vi "vision messing around.vi"() -> ()   [LabVIEW 2010]
panel:
  out "Image Out 3":T1(plugin-control)
  out "Image Out 2":T1(plugin-control)
  in  "Stop (F)":bool
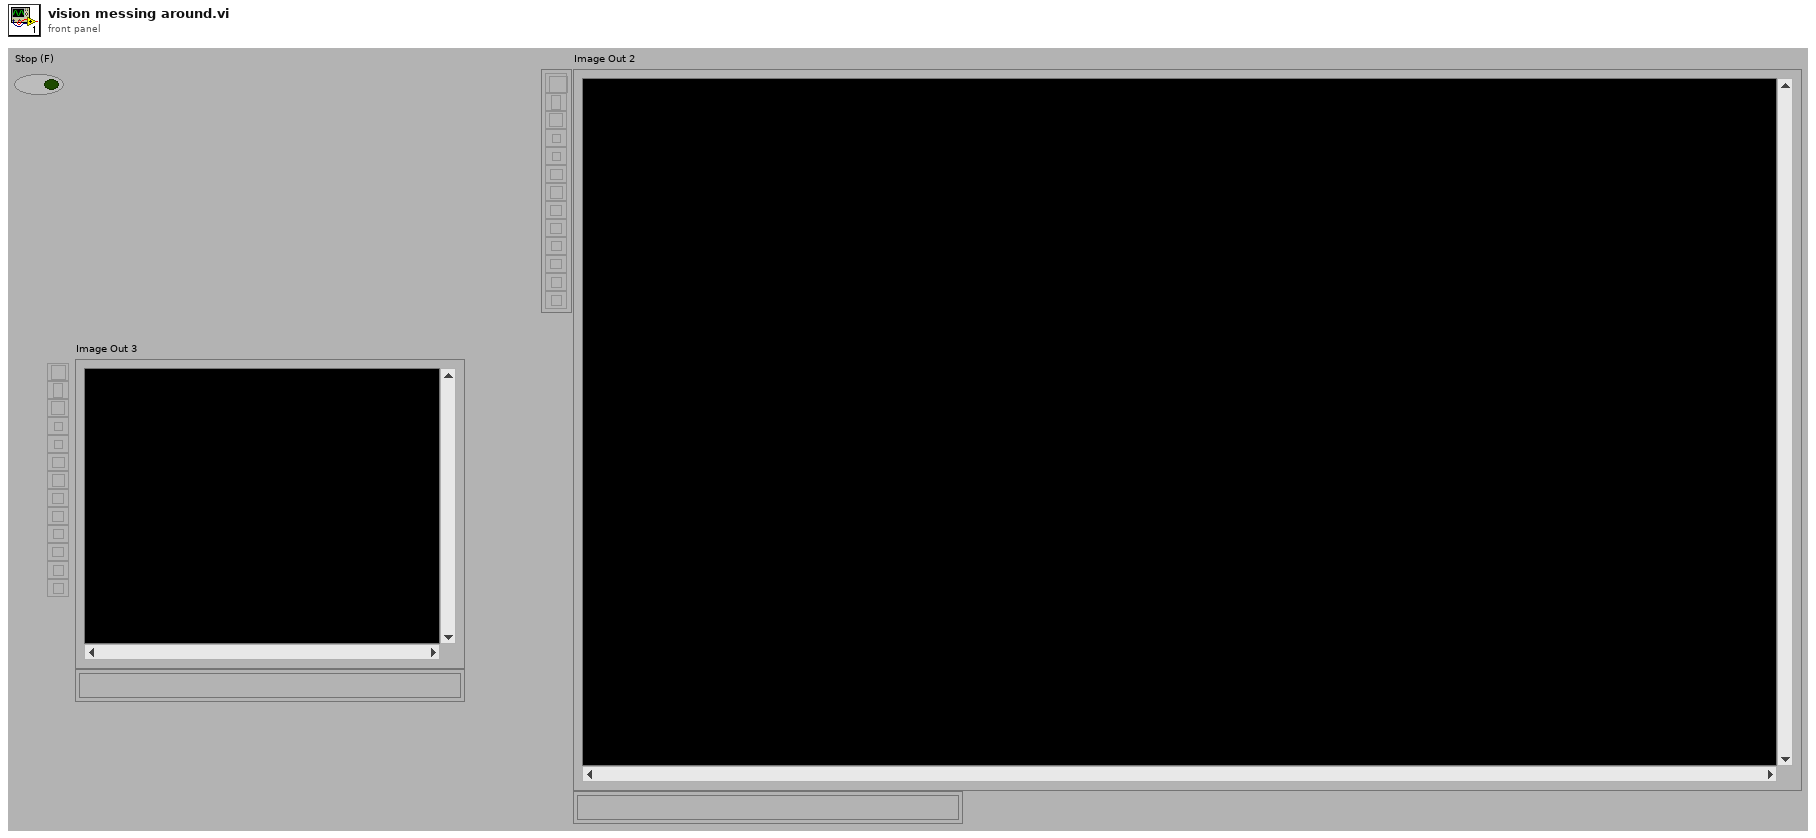
[diagram p1: front panel]
types:
  T1 = typedef "IMAQ Image.ctl" = refnum<image>
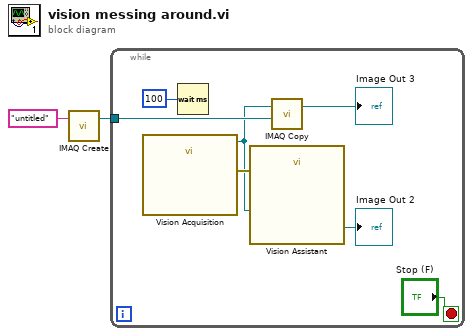
[diagram p0: block diagram]
diagram:
  n1 = call "IMAQ Create"("Image Name"="untitled") -> ("New Image"=w1:T1)  [unwired: 4 in, 1 out]
  n2 = while {
    tunnel: w1 -> [w7]
    stop <- "Stop (F)" stop-if-true
    n3 = call "Vision Acquisition"() -> ("Image Out"=w6:T1, "error out"=w9:errorcluster)  [unwired: 26 in]
    n4 = Wait (ms)(milliseconds to wait=u32 100) -> ()  [unwired: 1 out]
    n5 = call "Vision Assistant"("Image In"=w6, "error in"=w9) -> ("Image Out"=→"Image Out 2":T1)  [unwired: 24 in, 1 out]
    n6 = call "IMAQ Copy"("Image Dst"=w7, "Image Src"=w6) -> ("Image Dst Out"=→"Image Out 3":T1)  [unwired: 4 in, 1 out]
  }
